vi "SEA_9811_RT_Driver_Tester.vi"() -> ()   [LabVIEW 2012]
uses:
  Typdefs/SEA9811_RT_conf_cluster.ctl
  <vilib>/userdefined/High Color/nirio_resource_hc.ctl
  FPGA/SEA-9811_ReceiverAndTransmitter/SubVIs/SEA-9811_ReceiverAndTransmitter_RCR.ctl
  FPGA/SEA-9811_ReceiverAndTransmitter/SubVIs/SEA-9811_ReceiverAndTransmitter_TCR.ctl
  FPGA/SEA-9811_ReceiverAndTransmitter/SubVIs/SEA-9811_ReceiverAndTransmitter_RSR.ctl
  Typdefs/ARINC word cluster.ctl
  Typdefs/ARINC word.ctl
  Typdefs/channel.ctl
  Typdefs/received word.ctl
  <vilib>/Platform/TimedLoop/XDataNode/timing_clust.ctl
  <vilib>/Platform/TimedLoop/XDataNode/nitl_modes.ctl
  <vilib>/Platform/TimedLoop/XDataNode/wakeup.ctl
  <vilib>/Platform/TimedLoop/XDataNode/XDataNode.xnode
  <vilib>/Platform/TimedLoop/XDataNode/XDNodeRunTimeDep.lvlib
panel:
  out "Channels":T1[](array[typedef]) {"Received Words"."word" format="%.0o"; "Received Words"."timestamp" format="%#.10g"}
  in  "ARINC word in":T3 {"ARINC word" format="%032b"}
  out "error out":errorcluster
  in  "stop 2":bool
  out "Receiver Status Register (RSR)":T5={"RSR0: FIFO channel 0 empty"=TRUE, "RSR1: FIFO channel 1 empty"=TRUE, "RSR2: FIFO channel 2 empty"=TRUE, "RSR3: FIFO channel 3 empty"=TRUE, "RSR4: FIFO channel 4 empty"=TRUE, "RSR5: FIFO channel 5 empty"=TRUE, "RSR6: FIFO channel 6 empty"=TRUE, "RSR7: FIFO channel 7 empty"=TRUE, "RSR8: FIFO channel 0 full"=FALSE, "RSR9: FIFO channel 1 full"=FALSE, "RSR10: FIFO channel 2 full"=FALSE, "RSR11: FIFO channel 3 full"=FALSE, "RSR12: FIFO channel 4 full"=FALSE, "RSR13: FIFO channel 5 full"=FALSE, "RSR14: FIFO channel 6 full"=FALSE, "RSR15: FIFO channel 7 full"=FALSE}
  out "DMA Overflow":bool
  in  "stop":bool
  in  "SEA9811_conf_cluster":T6={"FPGA resource name"="RIO0", "Rx ch conf (0..7)"=[{"Rx Channel Number (0..7)"=0, "Rx Label Filter"={"Label 00"=0, "Label 01"=0, "Label 02"=0, "Label 03"=0, "Label 04"=0, "Label 05"=0, "Label 06"=0, "Label 07"=0, "Label 08"=0, "Label 09"=0, "Label 10"=0, "Label 11"=0, "Label 12"=0, "Label 13"=0, "Label 14"=0, "Label 15"=0}, "Receiver Control Register (RCR)"={"RCR0: Data rate = ARINC 429 High-Speed (0) or Low-Speed (1)"=FALSE, "RCR1: not used"=FALSE, "RCR2: Label recognition for this channel enabled (1) or disabled (0)"=FALSE, "RCR3: Receiver channel disabled (1) or enabled (0)"=FALSE, "RCR4: Odd parity check for this channel enabled (1) or disabled (0"=FALSE, "RCR5: Receiver normal operation (1) or loopback mode (0)"=TRUE, "RCR6: Receiver Decoder disabled (0) or enabled (1) \n-> ARINC bits 10 and 9 must match RCR7 and RCR8"=FALSE, "RCR7: If receiver decoder is enabled (RCR6=1), \nthe ARINC bit 10 must match this bit"=FALSE, "RCR8: If receiver decoder is enabled (RCR6=1), \nthe ARINC bit 9 must match this bit"=FALSE, "RCR9: Label bit order for this channel non-reversed (1) \nor reversed (0)"=FALSE, "RCR10: not used"=FALSE, "RCR11: not used"=FALSE, "RCR12: not used"=FALSE, "RCR13: not used"=FALSE, "RCR14: not used"=FALSE, "RCR15: not used"=FALSE}}, {"Rx Channel Number (0..7)"=3, "Rx Label Filter"={"Label 00"=23, "Label 01"=34, "Label 02"=0, "Label 03"=0, "Label 04"=0, "Label 05"=0, "Label 06"=0, "Label 07"=0, "Label 08"=0, "Label 09"=0, "Label 10"=0, "Label 11"=0, "Label 12"=0, "Label 13"=0, "Label 14"=0, "Label 15"=0}, "Receiver Control Register (RCR)"={"RCR0: Data rate = ARINC 429 High-Speed (0) or Low-Speed (1)"=FALSE, "RCR1: not used"=FALSE, "RCR2: Label recognition for this channel enabled (1) or disabled (0)"=FALSE, "RCR3: Receiver channel disabled (1) or enabled (0)"=FALSE, "RCR4: Odd parity check for this channel enabled (1) or disabled (0"=FALSE, "RCR5: Receiver normal operation (1) or loopback mode (0)"=TRUE, "RCR6: Receiver Decoder disabled (0) or enabled (1) \n-> ARINC bits 10 and 9 must match RCR7 and RCR8"=FALSE, "RCR7: If receiver decoder is enabled (RCR6=1), \nthe ARINC bit 10 must match this bit"=FALSE, "RCR8: If receiver decoder is enabled (RCR6=1), \nthe ARINC bit 9 must match this bit"=FALSE, "RCR9: Label bit order for this channel non-reversed (1) \nor reversed (0)"=FALSE, "RCR10: not used"=FALSE, "RCR11: not used"=FALSE, "RCR12: not used"=FALSE, "RCR13: not used"=FALSE, "RCR14: not used"=FALSE, "RCR15: not used"=FALSE}}, {"Rx Channel Number (0..7)"=5, "Rx Label Filter"={"Label 00"=2, "Label 01"=3, "Label 02"=0, "Label 03"=0, "Label 04"=0, "Label 05"=0, "Label 06"=0, "Label 07"=0, "Label 08"=0, "Label 09"=0, "Label 10"=0, "Label 11"=0, "Label 12"=0, "Label 13"=0, "Label 14"=0, "Label 15"=0}, "Receiver Control Register (RCR)"={"RCR0: Data rate = ARINC 429 High-Speed (0) or Low-Speed (1)"=FALSE, "RCR1: not used"=FALSE, "RCR2: Label recognition for this channel enabled (1) or disabled (0)"=FALSE, "RCR3: Receiver channel disabled (1) or enabled (0)"=FALSE, "RCR4: Odd parity check for this channel enabled (1) or disabled (0"=FALSE, "RCR5: Receiver normal operation (1) or loopback mode (0)"=TRUE, "RCR6: Receiver Decoder disabled (0) or enabled (1) \n-> ARINC bits 10 and 9 must match RCR7 and RCR8"=FALSE, "RCR7: If receiver decoder is enabled (RCR6=1), \nthe ARINC bit 10 must match this bit"=FALSE, "RCR8: If receiver decoder is enabled (RCR6=1), \nthe ARINC bit 9 must match this bit"=FALSE, "RCR9: Label bit order for this channel non-reversed (1) \nor reversed (0)"=FALSE, "RCR10: not used"=FALSE, "RCR11: not used"=FALSE, "RCR12: not used"=FALSE, "RCR13: not used"=FALSE, "RCR14: not used"=FALSE, "RCR15: not used"=FALSE}}], "Transmitter Control Register (TCR)"={"TCR0: not used"=FALSE, "TCR1: not used"=FALSE, "TCR2: not used"=FALSE, "TCR3: Transmitter Parity Bit Enable: 32nd bit is parity (1) or data (0)"=FALSE, "TCR4: not used"=FALSE, "TCR5: not used"=FALSE, "TCR6: not used"=FALSE, "TCR7: not used"=FALSE, "TCR8: not used"=FALSE, "TCR9: Transmitter Parity Select: odd parity (0) or even parity (1)"=FALSE, "TCR10: Transmitter Data Rate: ARINC 429 high-speed (0) or low-speed (1)"=FALSE, "TCR11: ARINC Label Bit Order: label bit order reversed (0) or not reversed (1)"=FALSE, "TCR12: Disable Line Driver: normal operation (0) or transmitter disabled (1)"=FALSE, "TCR13: Tansmit whenever data is available in FIFO (1) or only start by instruction \"Enable Transmission\" (0)"=TRUE, "TCR14: not used"=FALSE, "TCR15: not used"=FALSE}, "Bitfile Path"=path "c:/9082_SEA_9811_9220_IOsim.lvbitx"}
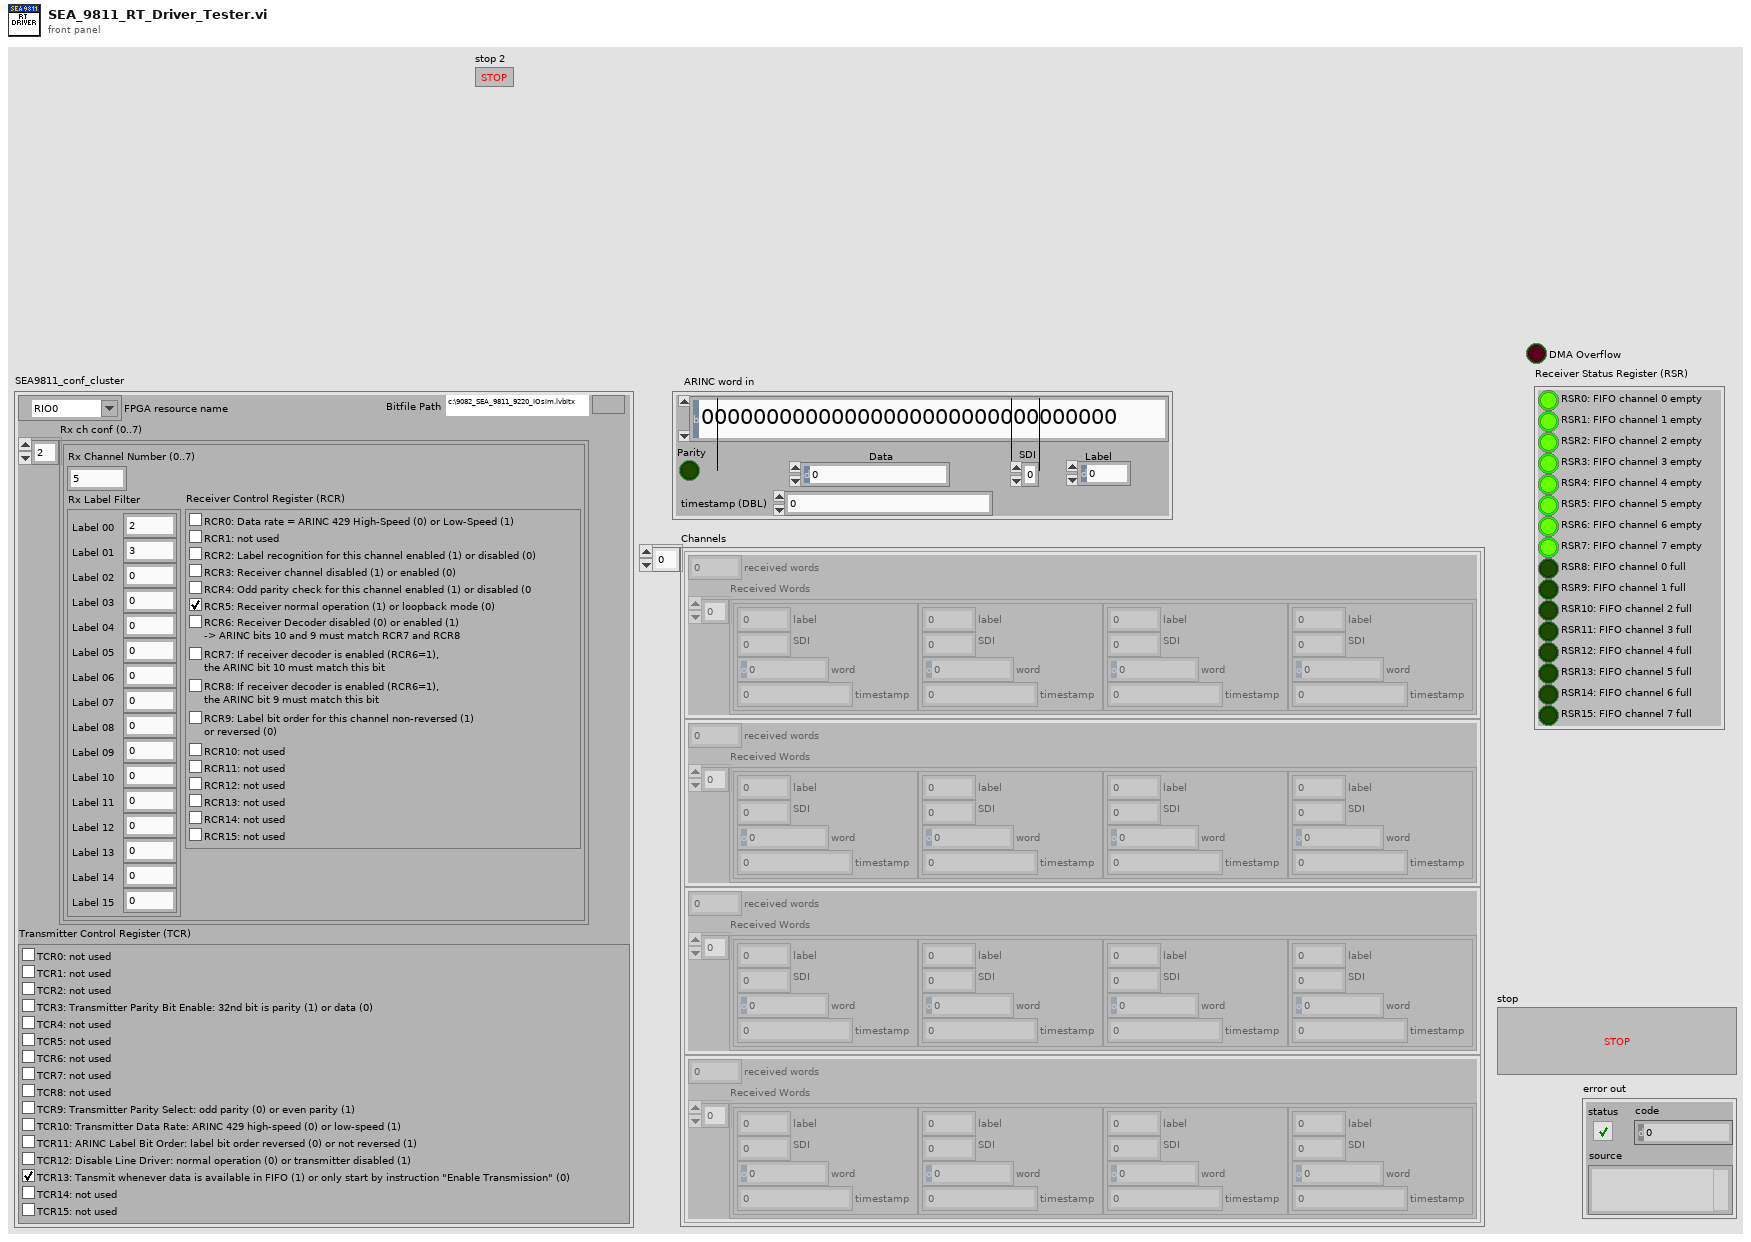
[diagram p1: front panel]
types:
  T1 = typedef "channel.ctl" = cluster{"received words":u32, "Received Words":T2[]}
  T2 = typedef "received word.ctl" = cluster{"label":u8, "SDI":u8, "word":u32, "timestamp":dbl}
  T3 = typedef "ARINC word cluster.ctl" = cluster{"ARINC word":T4, "Label":u8, "SDI":u8, "Data":u32, "Parity":bool, "timestamp (DBL)":dbl}
  T4 = typedef "ARINC word.ctl" = u32
  T5 = typedef "SEA-9811_ReceiverAndTransmitter_RSR.ctl" = cluster{"RSR0: FIFO channel 0 empty":bool, "RSR1: FIFO channel 1 empty":bool, "RSR2: FIFO channel 2 empty":bool, "RSR3: FIFO channel 3 empty":bool, "RSR4: FIFO channel 4 empty":bool, "RSR5: FIFO channel 5 empty":bool, "RSR6: FIFO channel 6 empty":bool, "RSR7: FIFO channel 7 empty":bool, "RSR8: FIFO channel 0 full":bool, "RSR9: FIFO channel 1 full":bool, "RSR10: FIFO channel 2 full":bool, "RSR11: FIFO channel 3 full":bool, "RSR12: FIFO channel 4 full":bool, "RSR13: FIFO channel 5 full":bool, "RSR14: FIFO channel 6 full":bool, "RSR15: FIFO channel 7 full":bool}
  T6 = typedef "SEA9811_RT_conf_cluster.ctl" = cluster{"FPGA resource name":T7, "Rx ch conf (0..7)":cluster{"Rx Channel Number (0..7)":u8, "Rx Label Filter":cluster{"Label 00":u8, "Label 01":u8, "Label 02":u8, "Label 03":u8, "Label 04":u8, "Label 05":u8, "Label 06":u8, "Label 07":u8, "Label 08":u8, "Label 09":u8, "Label 10":u8, "Label 11":u8, "Label 12":u8, "Label 13":u8, "Label 14":u8, "Label 15":u8}, "Receiver Control Register (RCR)":T8}[], "Transmitter Control Register (TCR)":T9, "Bitfile Path":path}
  T7 = typedef "nirio_resource_hc.ctl" = tag
  T8 = typedef "SEA-9811_ReceiverAndTransmitter_RCR.ctl" = cluster{"RCR0: Data rate = ARINC 429 High-Speed (0) or Low-Speed (1)":bool, "RCR1: not used":bool, "RCR2: Label recognition for this channel enabled (1) or disabled (0)":bool, "RCR3: Receiver channel disabled (1) or enabled (0)":bool, "RCR4: Odd parity check for this channel enabled (1) or disabled (0":bool, "RCR5: Receiver normal operation (1) or loopback mode (0)":bool, "RCR6: Receiver Decoder disabled (0) or enabled (1) \n-> ARINC bits 10 and 9 must match RCR7 and RCR8":bool, "RCR7: If receiver decoder is enabled (RCR6=1), \nthe ARINC bit 10 must match this bit":bool, "RCR8: If receiver decoder is enabled (RCR6=1), \nthe ARINC bit 9 must match this bit":bool, "RCR9: Label bit order for this channel non-reversed (1) \nor reversed (0)":bool, "RCR10: not used":bool, "RCR11: not used":bool, "RCR12: not used":bool, "RCR13: not used":bool, "RCR14: not used":bool, "RCR15: not used":bool}
  T9 = typedef "SEA-9811_ReceiverAndTransmitter_TCR.ctl" = cluster{"TCR0: not used":bool, "TCR1: not used":bool, "TCR2: not used":bool, "TCR3: Transmitter Parity Bit Enable: 32nd bit is parity (1) or data (0)":bool, "TCR4: not used":bool, "TCR5: not used":bool, "TCR6: not used":bool, "TCR7: not used":bool, "TCR8: not used":bool, "TCR9: Transmitter Parity Select: odd parity (0) or even parity (1)":bool, "TCR10: Transmitter Data Rate: ARINC 429 high-speed (0) or low-speed (1)":bool, "TCR11: ARINC Label Bit Order: label bit order reversed (0) or not reversed (1)":bool, "TCR12: Disable Line Driver: normal operation (0) or transmitter disabled (1)":bool, "TCR13: Tansmit whenever data is available in FIFO (1) or only start by instruction \"Enable Transmission\" (0)":bool, "TCR14: not used":bool, "TCR15: not used":bool}
  T10 = typedef "SEA9811_RT_data_cluster.ctl" = cluster{"FPGA VI Reference":T11, "Channels":T1[], "FPGA FP":T12}
  T11 = typedef "FPGA ref.ctl" = refnum<k20>
  T12 = typedef "SEA9811_FPGA_FP_Addresses.ctl" = cluster{"FPGA Interface Base on":refnum<class "FPGA Interface Base.lvclass">, "FPGA Session":u32, "RT time (ns)":u32, "DMA Overflow":u32, "Elements in FIFO":u32, "Rx Status":u32, "Rx Data (FIFO)":u32}
  T13 = typedef "XDNodeRunTimeDep.lvlib/timing_clust.ctl" = cluster{"Expected End [f-1]":u64, "Actual End [f-1]":u64, "Finished Late? [f-1]":bool, "Expected End [i-1]":u64, "Actual End [i-1]":u64, "Finished Late? [i-1]":bool, "Expected Start [i]":u64, "Actual Start [i]":u64, "Expected Start [f]":u64, "Actual Start [f]":u64, "Source Name":string, "Structure Name":string, "Period":i64, "Deadline":i64, "Offset":i64, "Start":i64, "Priority":i32, "Timeout":i32, "Mode":T14, "Wakeup Reason":T15, "Error":errorcluster, "Source Type":string, "Secondary Source Type":string, "Global End Time":u64, "Global Start Time":u64, "Frame Duration":u64, "Iteration Duration":u64, "Assigned CPU":i32, "I/O Scan Engine Mode":u32}
  T14 = typedef "XDNodeRunTimeDep.lvlib/nitl_modes.ctl" = enum32{"No Change", "Process missed periods, maintain original phase", "Discard missed periods, maintain original phase", "Process missed periods, ignore original phase", "Discard missed periods, ignore original phase"}
  T15 = typedef "XDNodeRunTimeDep.lvlib/wakeup.ctl" = enum32{"Normal", "Aborted", "Asynchronous wakeup", "Timing source error", "Timed loop error", "Timeout"}
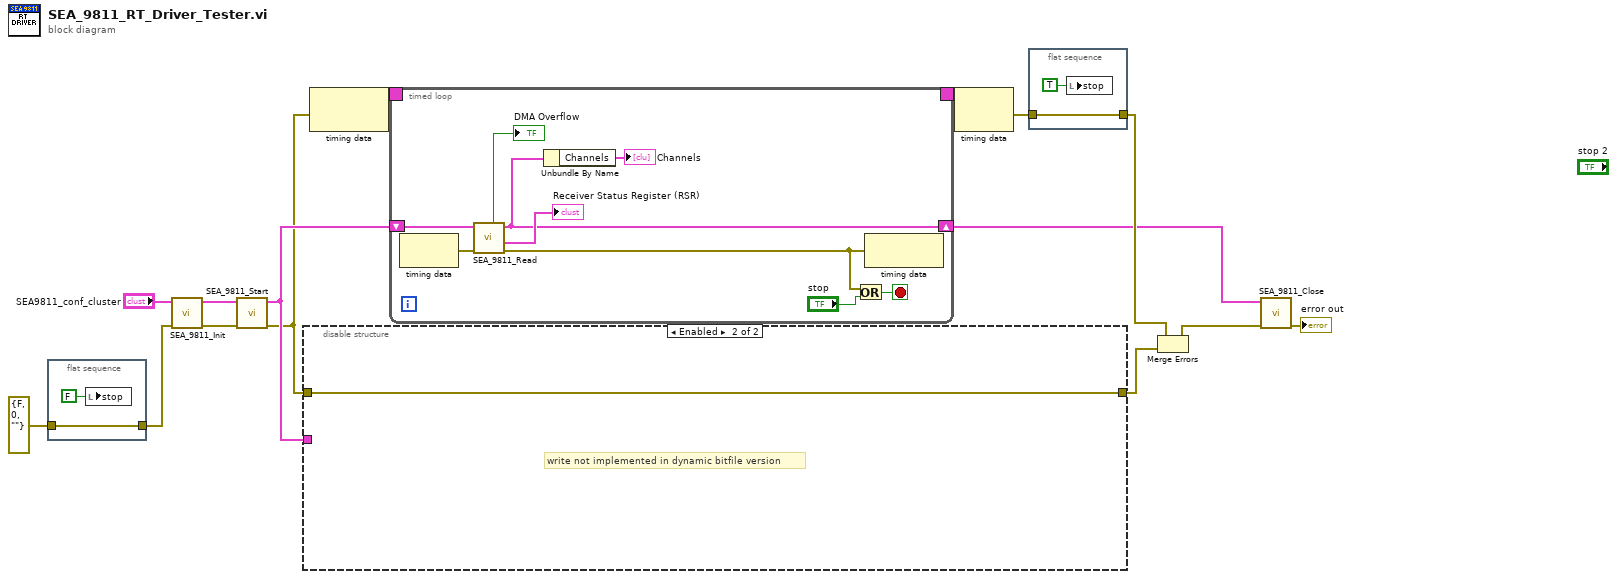
[diagram p0: block diagram]
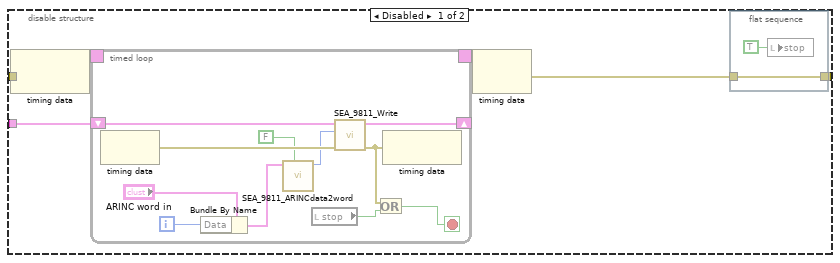
[diagram p2: hidden frame]
diagram:
  n1 = flat-sequence {
    tunnel: errorcluster {"status"=FALSE, "code"=0, "source"=""} ("error in") -> [w16]
    tunnel: [w16] -> w8
    frame #0 {
      n2 = local write "stop"(FALSE ("stop")) -> ()
    }
  }
  n3 = call "SEA_9811_Init.vi"("error in"=w8, "SEA9811_conf_cluster"="SEA9811_conf_cluster") -> ("error out"=w14:errorcluster, "SEA9811_RT_data out"=w1:T10)  [unwired: 8 in]
  n4 = call "SEA_9811_Start.vi"("error in (no error)"=w14, "SEA9811_RT_data in"=w1) -> ("error out"=w10:errorcluster, "SEA9811_RT_data out"=w13:T10)  [unwired: 8 in]
  n5 = disable-structure shown="Enabled" {
    disable-tunnel: w13 -> [w21 _]
    disable-tunnel: w10 -> [w20 w47]
    disable-tunnel: [w18 w47] -> w5
    frame Disabled {
      n6 = node-c288(w20) -> (w23:T13)
      n7 = timed-loop {
        timing: w23 -> [_]
        timing-out: [_] -> w22
        shift-right: [w29] -> _
        shift-left: w21 -> [w34]
        i -> [w27]
        stop <- w30 stop-if-true
        n8 = node-c288() -> (w33:errorcluster)  [unwired: 1 in]
        n9 = Bundle By Name(cluster="ARINC word in", "Data"=w27) -> (w25:T3)
        n10 = call "SEA_9811_ARINCdata2word.vi"("Reverse label bits"=FALSE, "ARINC word in"=w25) -> ("ARINC word out"=w28:T4)  [unwired: 8 in, 1 out]
        n11 = local read "stop"() -> (w32:bool)
        n12 = call "SEA_9811_Write.vi"("error in (no error)"=w33, "Tx Data"=w28, "SEA9811_RT_data in"=w34) -> ("error out"=w31:errorcluster, "SEA9811_RT_data out"=w29:T10)  [unwired: 7 in]
        n13 = Or(x=w31, y=w32) -> (x .or. y?=w30:bool)
        n14 = node-c288(w31) -> ()  [unwired: 1 out]
      }
      n15 = node-c288(w22) -> (w19:errorcluster)
      n16 = flat-sequence {
        tunnel: w19 -> [w45]
        tunnel: [w45] -> w18
        frame #0 {
          n17 = local write "stop"(TRUE ("stop")) -> ()
        }
      }
    }
    frame Enabled {
      # "write not implemented in dynamic bitfile version"
    }
  }
  n18 = node-c288(w10) -> (w12:T13)
  n19 = timed-loop {
    timing: w12 -> [_]
    timing-out: [_] -> w11
    shift-right: [w48] -> w3
    shift-left: w13 -> [w56]
    stop <- w53 stop-if-true
    n20 = node-c288() -> (w55:errorcluster)  [unwired: 1 in]
    n21 = call "SEA_9811_Read.vi"("error in (no error)"=w55, "SEA9811_RT_data in"=w56) -> ("error out"=w50:errorcluster, "Receiver Status Register (RSR)"=→"Receiver Status Register (RSR)":T5, "SEA9811_RT_data out"=w48:T10, "DMA Overflow"=→"DMA Overflow":bool)  [unwired: 6 in]
    n22 = Unbundle By Name(w48) -> ("Channels"=→"Channels":T1[])
    n23 = Or(x=w50, y="stop") -> (x .or. y?=w53:bool)
    n24 = node-c288(w50) -> ()  [unwired: 1 out]
  }
  n25 = node-c288(w11) -> (w7:errorcluster)
  n26 = flat-sequence {
    tunnel: w7 -> [w62]
    tunnel: [w62] -> w6
    frame #0 {
      n27 = local write "stop"(TRUE ("stop")) -> ()
    }
  }
  n28 = Merge Errors(w6, w5) -> (w4:errorcluster)
  n29 = call "SEA_9811_Close.vi"("error in (no error)"=w4, "SEA9811_RT_data in"=w3) -> ("error out"=→"error out":errorcluster)  [unwired: 9 in]
